vi "humanDetect.vi"(0 "KinectSensor References in":T10, 5 "Tracker":T8, 7 "colour mode (T = dist, F = sphere)":bool, 9 "Operation Mode":T9 items=["TeleOp", "Desperate", "ColourMatch"], 11 "Error In":errorcluster, 12 "Reference Colour":u32(colorbox)) -> (1 "Body Data":T1[](array[typedef]), 3 "index":i32, 4 "KinectSensor References":T10, 6 "Joint Position":T11, 10 "Image":T8(plugin-control), 13 "Averaged Colour":u32(colorbox), 14 "istracked":bool, 15 "Error Out":errorcluster)   [LabVIEW 2013]
uses:
  <vilib>/MakerHub/KinectOne/Private/Type Defs/KinectSensor References.ctl
  Microsoft.Kinect
  C:/Program Files (x86)/National Instruments/LabVIEW 2013/vi.lib/MakerHub/KinectOne/Private/Libs/BodyFrameDataInterface.dll
  Program Files (x86)/National Instruments/LabVIEW 2013/vi.lib/MakerHub/KinectOne/Private/Libs/BodyFrameDataInterface.dll
  <vilib>/vision/Image Controls.llb/IMAQ Image.ctl
  <vilib>/MakerHub/KinectOne/Private/Type Defs/Joint Position.ctl
  operationModes.ctl
  <vilib>/MakerHub/KinectOne/Private/Type Defs/BodyData.ctl
  <vilib>/MakerHub/KinectOne/Private/Type Defs/ClippedEdges.ctl
  <vilib>/MakerHub/KinectOne/Private/Type Defs/HandLeftConfidence.ctl
  <vilib>/MakerHub/KinectOne/Private/Type Defs/HandLeftState.ctl
  <vilib>/MakerHub/KinectOne/Private/Type Defs/HandRightConfidence.ctl
  <vilib>/MakerHub/KinectOne/Private/Type Defs/HandRightState.ctl
  <vilib>/MakerHub/KinectOne/Private/Type Defs/LeanTrackingState.ctl
  ColorMatch.ctl
  <vilib>/MakerHub/KinectOne/Private/Type Defs/JointType.ctl
  <vilib>/MakerHub/KinectOne/Private/kinectRead [ColorFrame].vi
  <vilib>/MakerHub/KinectOne/Private/kinectRead [BodyFrame].vi
  <vilib>/MakerHub/KinectOne/KinectOne.lvlib
panel:
  in  "alpha":dbl(slide)=0.7 scale=0.0..1.0
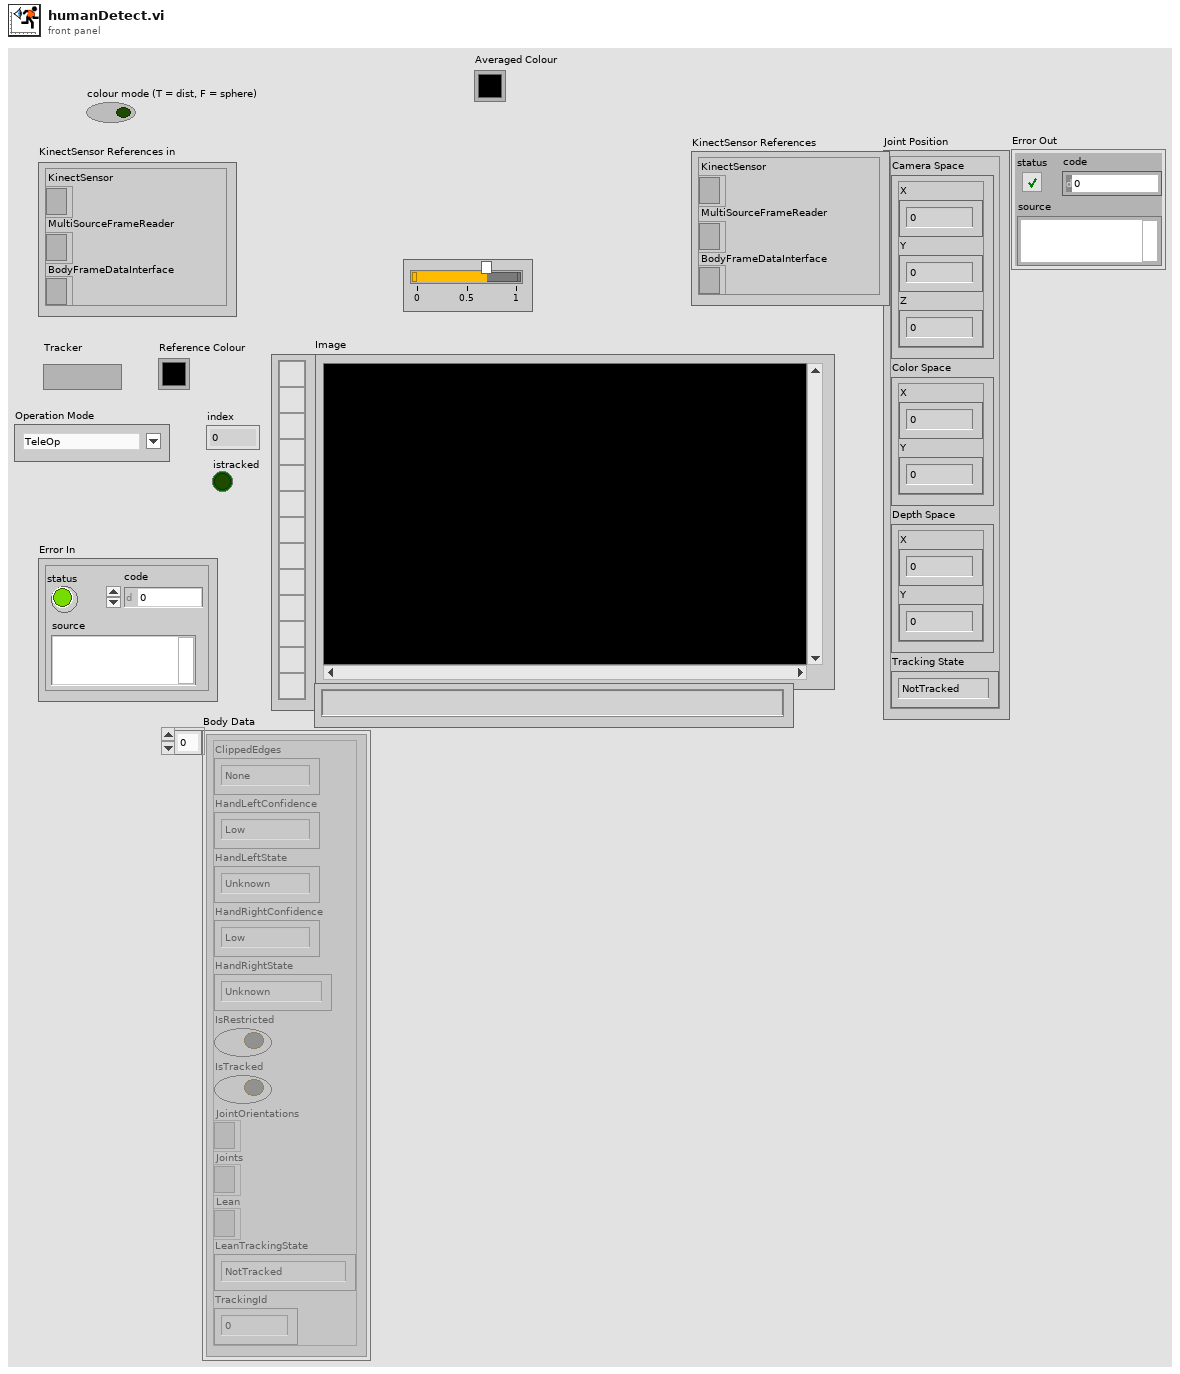
[diagram p1: front panel]
types:
  T1 = typedef "KinectOne.lvlib/BodyData.ctl" = cluster{"ClippedEdges":T2, "HandLeftConfidence":T3, "HandLeftState":T4, "HandRightConfidence":T5, "HandRightState":T6, "IsRestricted":bool, "IsTracked":bool, "JointOrientations":refnum<k24>, "Joints":refnum<k24>, "Lean":refnum<k24>, "LeanTrackingState":T7, "TrackingId":u64}
  T2 = typedef "KinectOne.lvlib/ClippedEdges.ctl" = enum16{"None", "Right", "Left", "Top", "Bottom"}
  T3 = typedef "KinectOne.lvlib/HandLeftConfidence.ctl" = enum16{"Low", "High"}
  T4 = typedef "KinectOne.lvlib/HandLeftState.ctl" = enum16{"Unknown", "NotTracked", "Open", "Closed", "Lasso"}
  T5 = typedef "KinectOne.lvlib/HandRightConfidence.ctl" = enum16{"Low", "High"}
  T6 = typedef "KinectOne.lvlib/HandRightState.ctl" = enum16{"Unknown", "NotTracked", "Open", "Closed", "Lasso"}
  T7 = typedef "KinectOne.lvlib/LeanTrackingState.ctl" = enum16{"NotTracked", "Inferred", "Tracked"}
  T8 = typedef "IMAQ Image.ctl" = refnum<image>
  T9 = typedef "operationModes.ctl" = u16
  T10 = typedef "KinectOne.lvlib/KinectSensor References.ctl" = cluster{"KinectSensor":refnum<k24>, "MultiSourceFrameReader":refnum<k24>, "BodyFrameDataInterface":refnum<k24>}
  T11 = typedef "KinectOne.lvlib/Joint Position.ctl" = cluster{"Camera Space":cluster{"X":dbl, "Y":dbl, "Z":dbl}, "Color Space":cluster{"X":dbl, "Y":dbl}, "Depth Space":cluster{"X":dbl, "Y":dbl}, "Tracking State":enum16{"NotTracked", "Inferred", "Tracked"}}
  T12 = typedef "KinectOne.lvlib/JointType.ctl" = enum16{"SpineBase", "SpineMid", "Neck", "Head", "ShoulderLeft", "ElbowLeft", "WristLeft", "HandLeft", "ShoulderRight", "ElbowRight", "WristRight", "HandRight", "HipLeft", "KneeLeft", "AnkleLeft", "FootLeft", "HipRight", "KneeRight", "AnkleRight", "FootRight", "SpineShoulder", "HandTipLeft", "ThumbLeft", "HandTipRight", "ThumbRight"}
  T13 = typedef "ColorMatch.ctl" = cluster{"weighted score":dbl, "index":i32, "Color Box":u32}
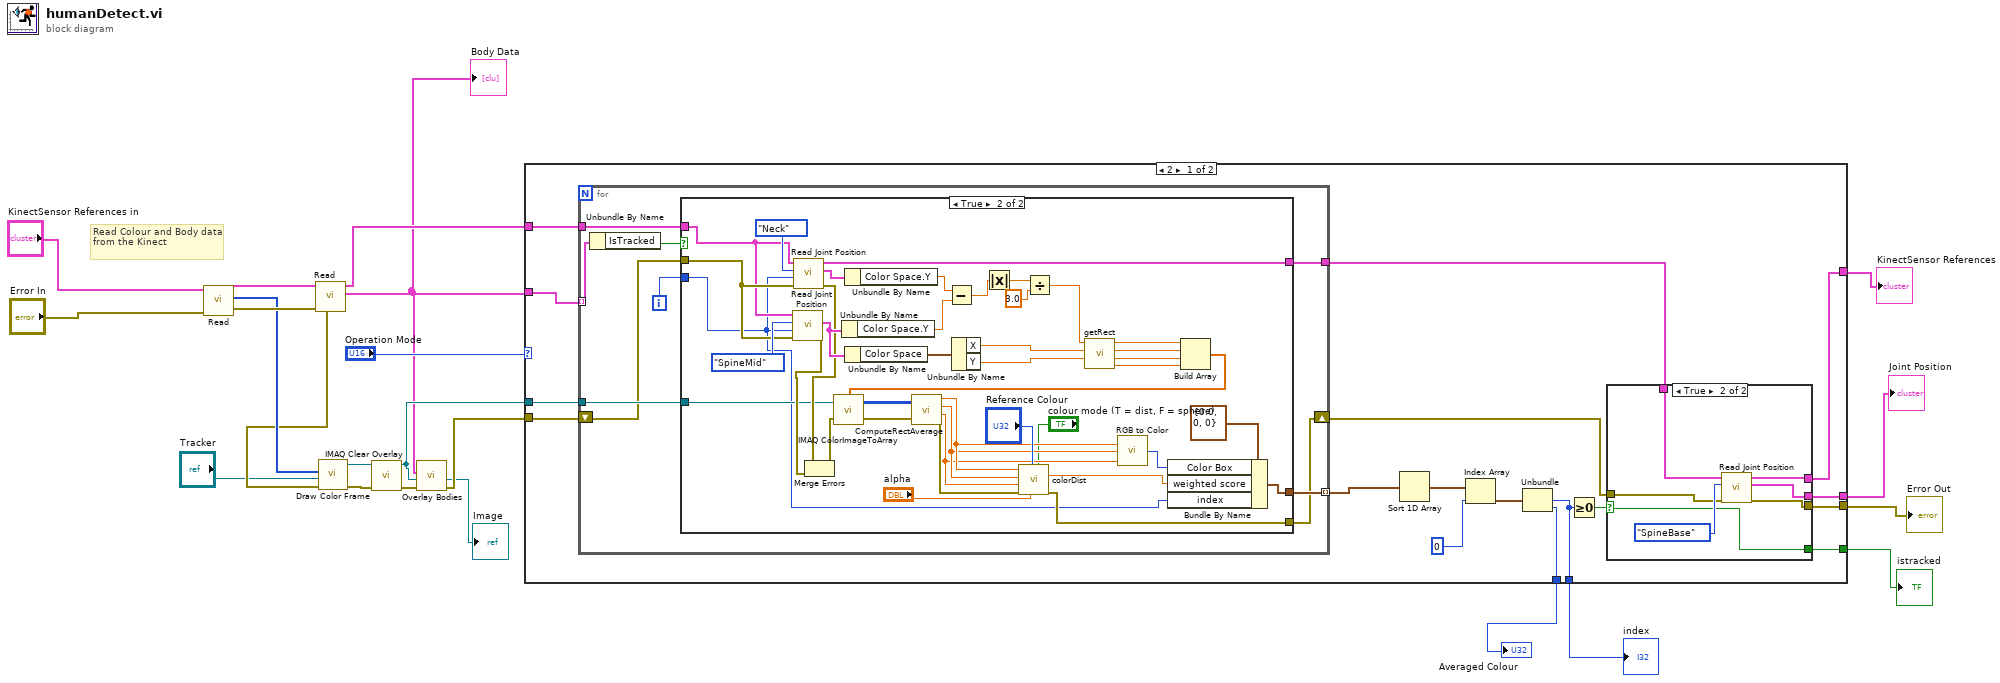
[diagram p0: block diagram]
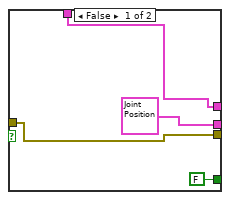
[diagram p2: hidden frame]
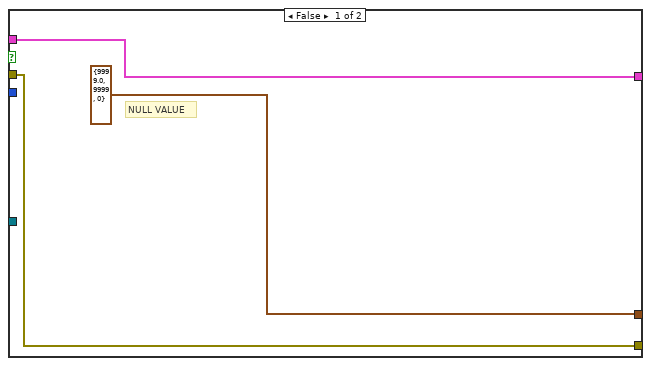
[diagram p3: hidden frame]
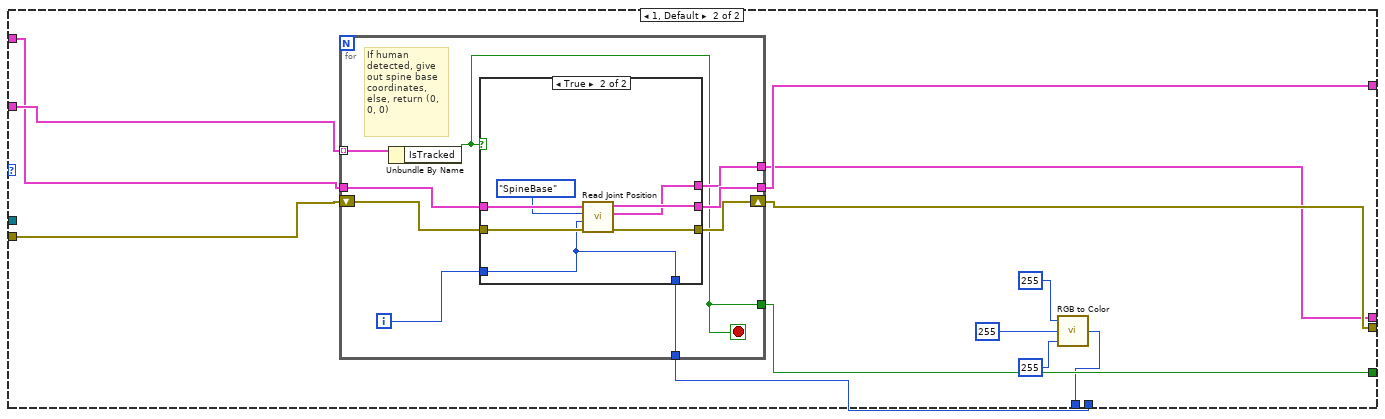
[diagram p4: hidden frame]
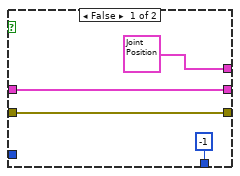
[diagram p5: hidden frame]
diagram:
  # "Read Colour and Body data from the Kinect"
  n1 = call-poly <vilib>:"Read.vi"("Error In"="Error In", "KinectSensor References in"="KinectSensor References in") -> ("Error Out"=w22:errorcluster, "frameData"=w19:u32[], "KinectSensor References out"=w21:T10)  [unwired: 7 in]
  n2 = call-poly <vilib>:"Read.vi"("error in (no error)"=w22, "KinectSensor References in"=w21) -> ("error out"=w18:errorcluster, "Body Data"=w2:T1[], "KinectSensor References out"=w10:T10)  [unwired: 7 in]
  "Body Data" <- w2
  n3 = call <vilib>:"Draw Color Frame.vi"("Error In"=w18, "U32 Array"=w19, "Image"="Tracker") -> ("Error Out"=w16:errorcluster, "Image Out"=w13:T8)  [unwired: 7 in]
  n4 = call "IMAQ Clear Overlay"("error in (no error)"=w16, "Image"=w13) -> ("error out"=w15:errorcluster, "Image Out"=w12:T8)  [unwired: 8 in]
  n5 = call <vilib>:"Overlay Bodies.vi"("Error In"=w15, "Image"=w12, "Body Data"=w2) -> ("Error Out"=w11:errorcluster, "Image Out"=→"Image":T8)  [unwired: 7 in]
  n6 = case shown="2" "Operation Mode" {
    tunnel: w12 -> [w33 _]
    tunnel: w11 -> [w32 w107]
    tunnel: w10 -> [w31 w113]
    tunnel: [w30 w110] -> w9
    tunnel: [w29 w109] -> w8
    tunnel: [w27 w111] -> w7
    tunnel: w2 -> [w25 w114]
    tunnel: [w26 w112] -> w6
    tunnel: [w24 w108] -> w5
    tunnel: [w23 w103] -> w1
    frame 2 {
      n7 = for {
        tunnel: [w57] -> w35
        tunnel: [w56] -> w39 mode=indexing
        tunnel: w33 -> [w55]
        shift-right: [w53] -> w28
        shift-left: w32 -> [w54]
        tunnel: w31 -> [w52]
        tunnel: w25 -> [w51] mode=indexing
        i -> [w58]
        n8 = Unbundle By Name(w51) -> ("IsTracked"=w59:bool)
        n9 = case shown="True" w59 {
          tunnel: w58 -> [_ w71]
          tunnel: [w60 w100] -> w57
          tunnel: [T13 {"weighted score"=9999.0, "index"=9999, "Color Box"=0} w70] -> w56
          tunnel: w55 -> [_ w74]
          tunnel: w54 -> [w61 w86]
          tunnel: [w61 w80] -> w53
          tunnel: w52 -> [w60 w79]
          frame False {
            # "NULL VALUE"
          }
          frame True {
            n10 = call <vilib>:"Read Joint Position.vi"("Error In"=w86, "Body Index"=w71, "JointType"=JointType."SpineMid", "KinectSensor References"=w79) -> ("Error Out"=w83:errorcluster, "Joint Position"=w87:T11)  [unwired: 4 in, 2 out]
            n11 = call <vilib>:"Read Joint Position.vi"("Error In"=w86, "Body Index"=w71, "JointType"=JointType."Neck", "KinectSensor References"=w79) -> ("Error Out"=w84:errorcluster, "Joint Position"=w99:T11, "KinectSensor References"=w100:T10)  [unwired: 4 in, 1 out]
            n12 = Merge Errors(w84, w83) -> (w85:errorcluster)
            n13 = Unbundle By Name(w87) -> ("Color Space.Y"=w97:dbl)
            n14 = Unbundle By Name(w99) -> ("Color Space.Y"=w98:dbl)
            n15 = Unbundle By Name(w87) -> ("Color Space"=w96:cluster{"X":dbl, "Y":dbl})
            n16 = Subtract(x=w98, y=w97) -> (x-y=w76:dbl)
            n17 = Unbundle By Name(w96) -> ("X"=w93:dbl, "Y"=w92:dbl)
            n18 = Absolute Value(x=w76) -> (abs(x)=w77:dbl)
            n19 = Divide(x=w77, y=3.0) -> (x/y=w94:dbl)
            n20 = call "getRect.vi"("Y"=w92, "X"=w93, "Offset"=w94) -> ("B"=w88:dbl, "R"=w89:dbl, "T"=w90:dbl, "L"=w91:dbl)  [unwired: 5 in]
            n21 = Build Array(w91, w90, w89, w88) -> (w73:dbl[])
            n22 = call "IMAQ ColorImageToArray"("Optional Rectangle"=w73, "Image"=w74, "error in (no error)"=w85) -> ("Image Pixels (U32)"=w75:u32[][], "error out"=w82:errorcluster)  [unwired: 1 in, 1 out]
            n23 = call "ComputeRectAverage.vi"("Error In"=w82, "Image Pixels (U32)"=w75) -> ("error IO"=w81:errorcluster, "Bavg"=w66:dbl, "Gavg"=w67:dbl, "Ravg"=w68:dbl)  [unwired: 1 in]
            n24 = call "colorDist.vi"("colour mode (T = dist, F = sphere)"="colour mode (T = dist, F = sphere)", "alpha"="alpha", "Reference Colour"="Reference Colour", "error in"=w81, "B"=w66, "G"=w67, "R"=w68) -> ("error out"=w80:errorcluster, "weighted score"=w72:dbl)  [unwired: 2 in]
            n25 = call <vilib>:"RGB to Color.vi"("B"=w66, "G"=w67, "R"=w68) -> ("Color"=w64:u32)
            n26 = Bundle By Name(cluster=T13 {"weighted score"=0.0, "index"=0, "Color Box"=0} ("Cluster"), "Color Box"=w64, "weighted score"=w72, "index"=w71) -> (w70:T13)
          }
        }
      }
      n27 = Sort 1D Array(array=w39) -> (sorted array=w38:T13[])
      n28 = Index Array(array=w38, index=0) -> (element=w36:T13)
      n29 = Unbundle(w36) -> ("index"=w24:i32, "Color Box"=w23:u32)  [unwired: 1 out]
      n30 = Greater Or Equal To 0?(x=w24) -> (x >= 0?=w34:bool)
      n31 = case shown="True" w34 {
        selector: w34 -> [_ w44]
        tunnel: w35 -> [w42 w50]
        tunnel: [w42 w48] -> w30
        tunnel: [T11 {"Camera Space"={"X"=0.0, "Y"=0.0, "Z"=0.0}, "Color Space"={"X"=0.0, "Y"=0.0}, "Depth Space"={"X"=0.0, "Y"=0.0}, "Tracking State"=enum."NotTracked"} ("Joint Position") w47] -> w29
        tunnel: w28 -> [w41 w46]
        tunnel: [w41 w45] -> w27
        tunnel: [FALSE ("Tracked?") w44] -> w26
        frame False {
        }
        frame True {
          n32 = call <vilib>:"Read Joint Position.vi"("Error In"=w46, "JointType"=JointType."SpineBase", "KinectSensor References"=w50) -> ("Error Out"=w45:errorcluster, "Joint Position"=w47:T11, "KinectSensor References"=w48:T10)  [unwired: 5 in, 1 out]
        }
      }
    }
    frame 1, Default {
      n33 = for {
        shift-right: [w118] -> w111
        shift-left: w107 -> [w119]
        tunnel: w114 -> [w123] mode=indexing
        tunnel: w113 -> [w122]
        tunnel: [w121] -> w110
        tunnel: [w120] -> w109
        tunnel: [w115] -> w112
        tunnel: [w116] -> w108
        i -> [w117]
        stop <- w115 stop-if-true
        # "If human detected, give out spine base coordinates,\nelse, return (0, 0, 0)"
        n34 = Unbundle By Name(w123) -> ("IsTracked"=w115:bool)
        n35 = case shown="True" w115 {
          tunnel: w122 -> [w127 w134]
          tunnel: [w127 w133] -> w121
          tunnel: [T11 {"Camera Space"={"X"=0.0, "Y"=0.0, "Z"=0.0}, "Color Space"={"X"=0.0, "Y"=0.0}, "Depth Space"={"X"=0.0, "Y"=0.0}, "Tracking State"=enum."NotTracked"} ("Joint Position") w131] -> w120
          tunnel: w119 -> [w125 w130]
          tunnel: [w125 w129] -> w118
          tunnel: w117 -> [_ w128]
          tunnel: [-1 w128] -> w116
          frame False {
          }
          frame True {
            n36 = call <vilib>:"Read Joint Position.vi"("Error In"=w130, "Body Index"=w128, "JointType"=JointType."SpineBase", "KinectSensor References"=w134) -> ("Error Out"=w129:errorcluster, "Joint Position"=w131:T11, "KinectSensor References"=w133:T10)  [unwired: 4 in, 1 out]
          }
        }
      }
      n37 = call <vilib>:"RGB to Color.vi"("B"=u8 255 ("R"), "G"=u8 255 ("R"), "R"=u8 255) -> ("Color"=w103:u32)
    }
  }
  "Joint Position" <- w8
  "KinectSensor References" <- w9
  "Error Out" <- w7
  "istracked" <- w6
  "index" <- w5
  "Averaged Colour" <- w1
